vi "Periodic Tasks.vi"(8 "error in":errorcluster) -> ()   [LabVIEW 2018]
doc: "This VI runs in parallel to other tasks. It can contain as many user-defined periodic loops as you need. These can carry out PID or other sorts of timed response."
uses:
  <vilib>/Rock Robotics/WPI/Solenoid/WPI_SolenoidValue.ctl
  <vilib>/Rock Robotics/WPI/ThirdParty/Phoenix-LabVIEW/Motor Controller/Controls/CTRE_Phoenix_MotorControl_ControlMode.ctl
  <vilib>/Rock Robotics/WPI/DriverStation/WPI_DriverStationRobotMode2.ctl
  ca579f97-49ab-43f2-8d57-79325bc44b91.vi
  49744297-d732-4f26-b9df-ea13e04ead65.vi
  0c7d2dc5-c582-4743-8fb3-b9c2bdc871ef.vi
  0ab41fdd-f005-4a41-8abb-d0c1aebc8839.vi
  eb1224c5-d191-4a5a-b208-f0176ff8254b.vi
  4d1e90e2-2e56-4cd0-9c54-8509fccd737b.vi
  fa0b2ed9-014b-4d02-a9e7-965de739ed34.vi
  3bc81077-0bee-49a4-9064-f6dc6ff34700.vi
  c6107473-3bbc-4d68-b130-33bb0f28684e.vi
  bc72f310-a025-467b-8a7d-9af20b832017.vi
  627df16c-e363-45ec-ab0c-cc0e3a3b33f7.vi
  ea05d6e2-4bc2-4863-96e4-0034388c650a.vi
  93672789-ce46-4bc6-a5b5-faff44e817a8.vi
  c8be7294-c6ee-427e-ae78-3199e8744a18.vi
  1c7609ed-6cb5-470b-bbb9-41d14296924d.vi
  50b6936b-a54e-4087-a151-83919d29fb22.vi
  efed0d96-a490-4904-9cbf-ad4873da1ad9.vi
  RobotStates.vi
  Robot Global Data.vi
  <vilib>/Rock Robotics/Network Tables/NT Write Number.vi
  RefNums_DriverStation.vi
  <vilib>/Rock Robotics/WPI/Utilities/WPI_GetSetVariantRefNum.vi
  RefNums_Actuators.vi
  <vilib>/Rock Robotics/WPI/Solenoid/WPI_SolenoidSetEnum.vi
  RefNums_Sensors.vi
  SensorReadings.vi
  Inputs_DriverStation.vi
panel:
  in  "Time in Error Band (ms)":u32=500
  in  "Error Band (in)":dbl=1.0
  in  "Max Down Power":dbl=-0.5 format="%#_13g"
  out "Sensor Loop (ms)":u32
  in  "Enable Plotting":bool
  out "Control Loop Time (ms)":u32
  out "PID Tracking":cluster{"Goal Wheel Position":dbl, dbl}(graph)={"Goal Wheel Position"=0.0, -90.17571233858979}
  out "Contribution Tracking":cluster{dbl, dbl, dbl}(graph)
  in  "N-Int":i32=25
  in  "N-Diff":i32=20
  in  "Kd":dbl=0.01
  in  "Ki":dbl=0.02
  in  "Kp":dbl=0.04
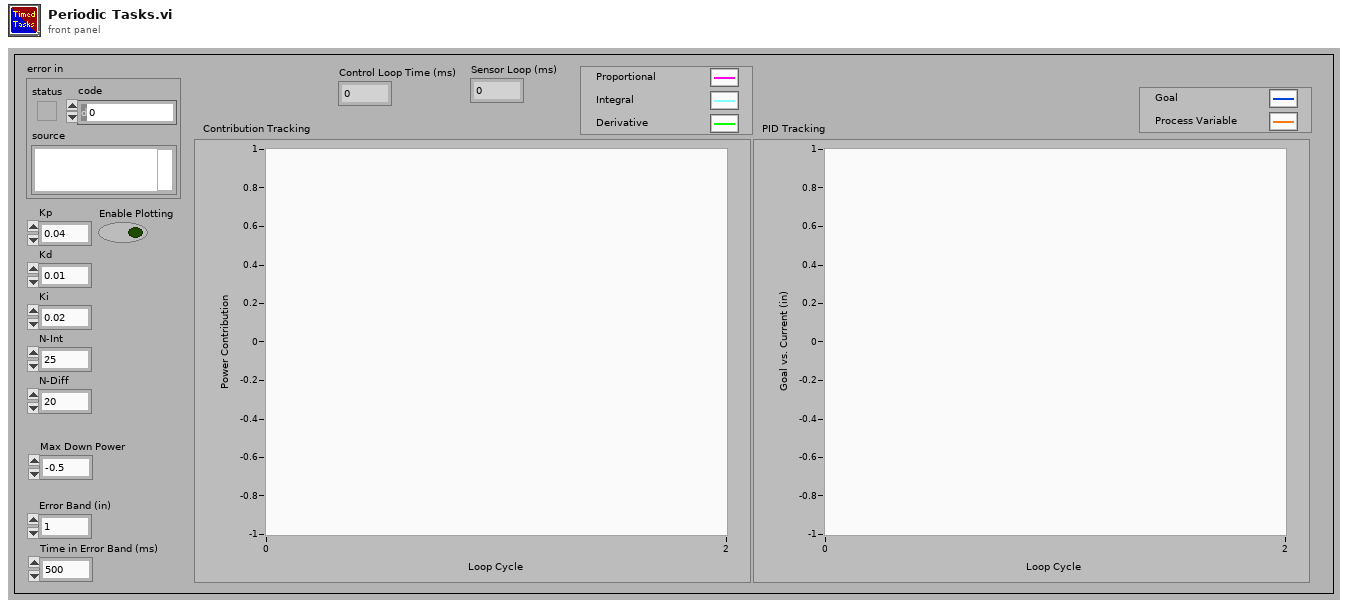
[diagram p1: front panel]
types:
  T1 = typedef "WPI_MotorControlDeviceRef.ctl" = cluster{"DeviceStatus":errorcluster, "Type":T2, "PWM":cluster{"PWM Channel":T3, "DeadBand":T4}, "CAN":cluster{"Device Number":u8, "SetOutput VI Ref":variant, "GetOutput VI Ref":variant, "Enable VI Ref":variant, "Disable VI Ref":variant, "Data":variant}, "Invert":bool, "DIO PWM":cluster{"PWM \"Enable\" Channel":T3, "DIOChannel":T5, "PWM Rate":dbl}}
  T2 = typedef "WPI_MotorControlType.ctl" = enum16{"PWM", "CAN", "DIO PWM"}
  T3 = typedef "FPGA_DIOPWMChannel.ctl" = enum8{"PWM 0", "PWM 1", "PWM 2", "PWM 3", "PWM 4", "PWM 5", "PWM 6", "PWM 7", "PWM 8", "PWM 9", "PWM MXP 0", "PWM MXP 1", "PWM MXP 2", "PWM MXP 3", "PWM MXP 4", "PWM MXP 5", "PWM MXP 6", "PWM MXP 7", "PWM MXP 8", "PWM MXP 9", "Invalid"}
  T4 = typedef "WPI_PWMDeadband.ctl" = cluster{"Name":string, "maxPositivePwm":i32, "minPositivePwm":i32, "centerPwm":i32, "maxNegativePwm":i32, "minNegativePwm":i32, "angularRange":u16}
  T5 = typedef "FPGA_DIOChannel.ctl" = enum8{"DIO 0", "DIO 1", "DIO 2", "DIO 3", "DIO 4", "DIO 5", "DIO 6", "DIO 7", "DIO 8", "DIO 9", "DIO MXP 0", "DIO MXP 1", "DIO MXP 2", "DIO MXP 3", "DIO MXP 4", "DIO MXP 5", "DIO MXP 6", "DIO MXP 7", "DIO MXP 8", "DIO MXP 9", "DIO MXP 10", "DIO MXP 11", "DIO MXP 12", "DIO MXP 13", "DIO MXP 14", "DIO MXP 15", "SPI Port CS1", "SPI Port CS2", "SPI Port CS3", "SPI Port MISO", "SPI Port MOSI", "Invalid"}
  T6 = typedef "WPI_SolenoidDevRef.ctl" = cluster{"DevStatus":errorcluster, "Pneumatics Control Module":u8, "Forward Solenoid Channel":T7, "Reverse Solenoid Channel":T7}
  T7 = typedef "WPI_SolenoidChannel.ctl" = enum8{"Solenoid 0", "Solenoid 1", "Solenoid 2", "Solenoid 3", "Solenoid 4", "Solenoid 5", "Solenoid 6", "Solenoid 7", "Invalid"}
  T8 = typedef "WPI_ServoDeviceRef.ctl" = cluster{"DeviceStatus":errorcluster, "PWM Channel":T3, "DeadBand":T4}
  T9 = typedef "WPI_RobotDriveDevRef.ctl" = cluster{"DevStatus":errorcluster, "Motors[]":T1[], "Square Inputs":bool, "Max Output":dbl}
  T10 = typedef "WPI_JoystickDevRef.ctl" = cluster{"Device":T11}
  T11 = typedef "WPI_JoystickDeviceEnum.ctl" = enum16{"USB 0", "USB 1", "USB 2", "USB 3", "USB 4", "USB 5"}
  T12 = typedef "WPI_CompressorDevRef.ctl" = cluster{"DevStatus":errorcluster, "Pneumatics Control Module":u8}
  T13 = typedef "WPI_AccelerometerDevRef.ctl" = cluster{"DevStatus":errorcluster, "Scaling":T14, "Analog Channels":T15, "I2C Bus":T17, "SPI Bus":T18, "Accel Range":T19, "ADXL Axes":T20, "Handle":i32, "Device Address":u8, "Accel Type":enum16{"Analog", "ADXL345 I2C", "ADXL345 SPI", "Internal", "ADXL362 SPI"}}
  T14 = typedef "WPI_AccelerometerScaling.ctl" = cluster{"Gain (VoltsPerG)":dbl, "Center Voltage":dbl}
  T15 = typedef "WPI_AccelerometerAnalogChannels.ctl" = cluster{"X-Axis":T16, "Y-Axis":T16, "Z-Axis":T16}
  T16 = typedef "FPGA_AIChannel.ctl" = enum8{"AI 0", "AI 1", "AI 2", "AI 3", "AI MXP 0", "AI MXP 1", "AI MXP 2", "AI MXP 3", "Invalid"}
  T17 = typedef "i2c_bus.ctl" = enum16{"I2C On-Board", "I2C MXP", "Invalid"}
  T18 = typedef "spi_bus.ctl" = enum16{"SPI On-Board, CS0", "SPI On-Board, CS1", "SPI On-Board, CS2", "SPI On-Board, CS3", "SPI MXP", "Invalid"}
  T19 = typedef "ADXL345 Range.ctl" = u8
  T20 = typedef "WPI_AccelerometerADXL345 Axes.ctl" = cluster{"X-Axis":bool, "Y-Axis":bool, "Z-Axis":bool}
  T21 = typedef "WPI_AnalogChannelDevRef.ctl" = cluster{"DevStatus":errorcluster, "Analog Channel":T16}
  T22 = typedef "WPI_DriverStationRobotMode2.ctl" = enum16{"Autonomous Disabled", "Autonomous Enabled", "Teleop Disabled", "Teleop Enabled", "Disconnected", "Finish", "Test Disabled", "Test Enabled", "Emergency Stopped"}
  T23 = typedef "CTRE_Phoenix_MotorControl_ControlMode.ctl" = u16
  T24 = typedef "WPI_SolenoidValue.ctl" = enum16{"Off", "On", "Forward", "Reverse"}
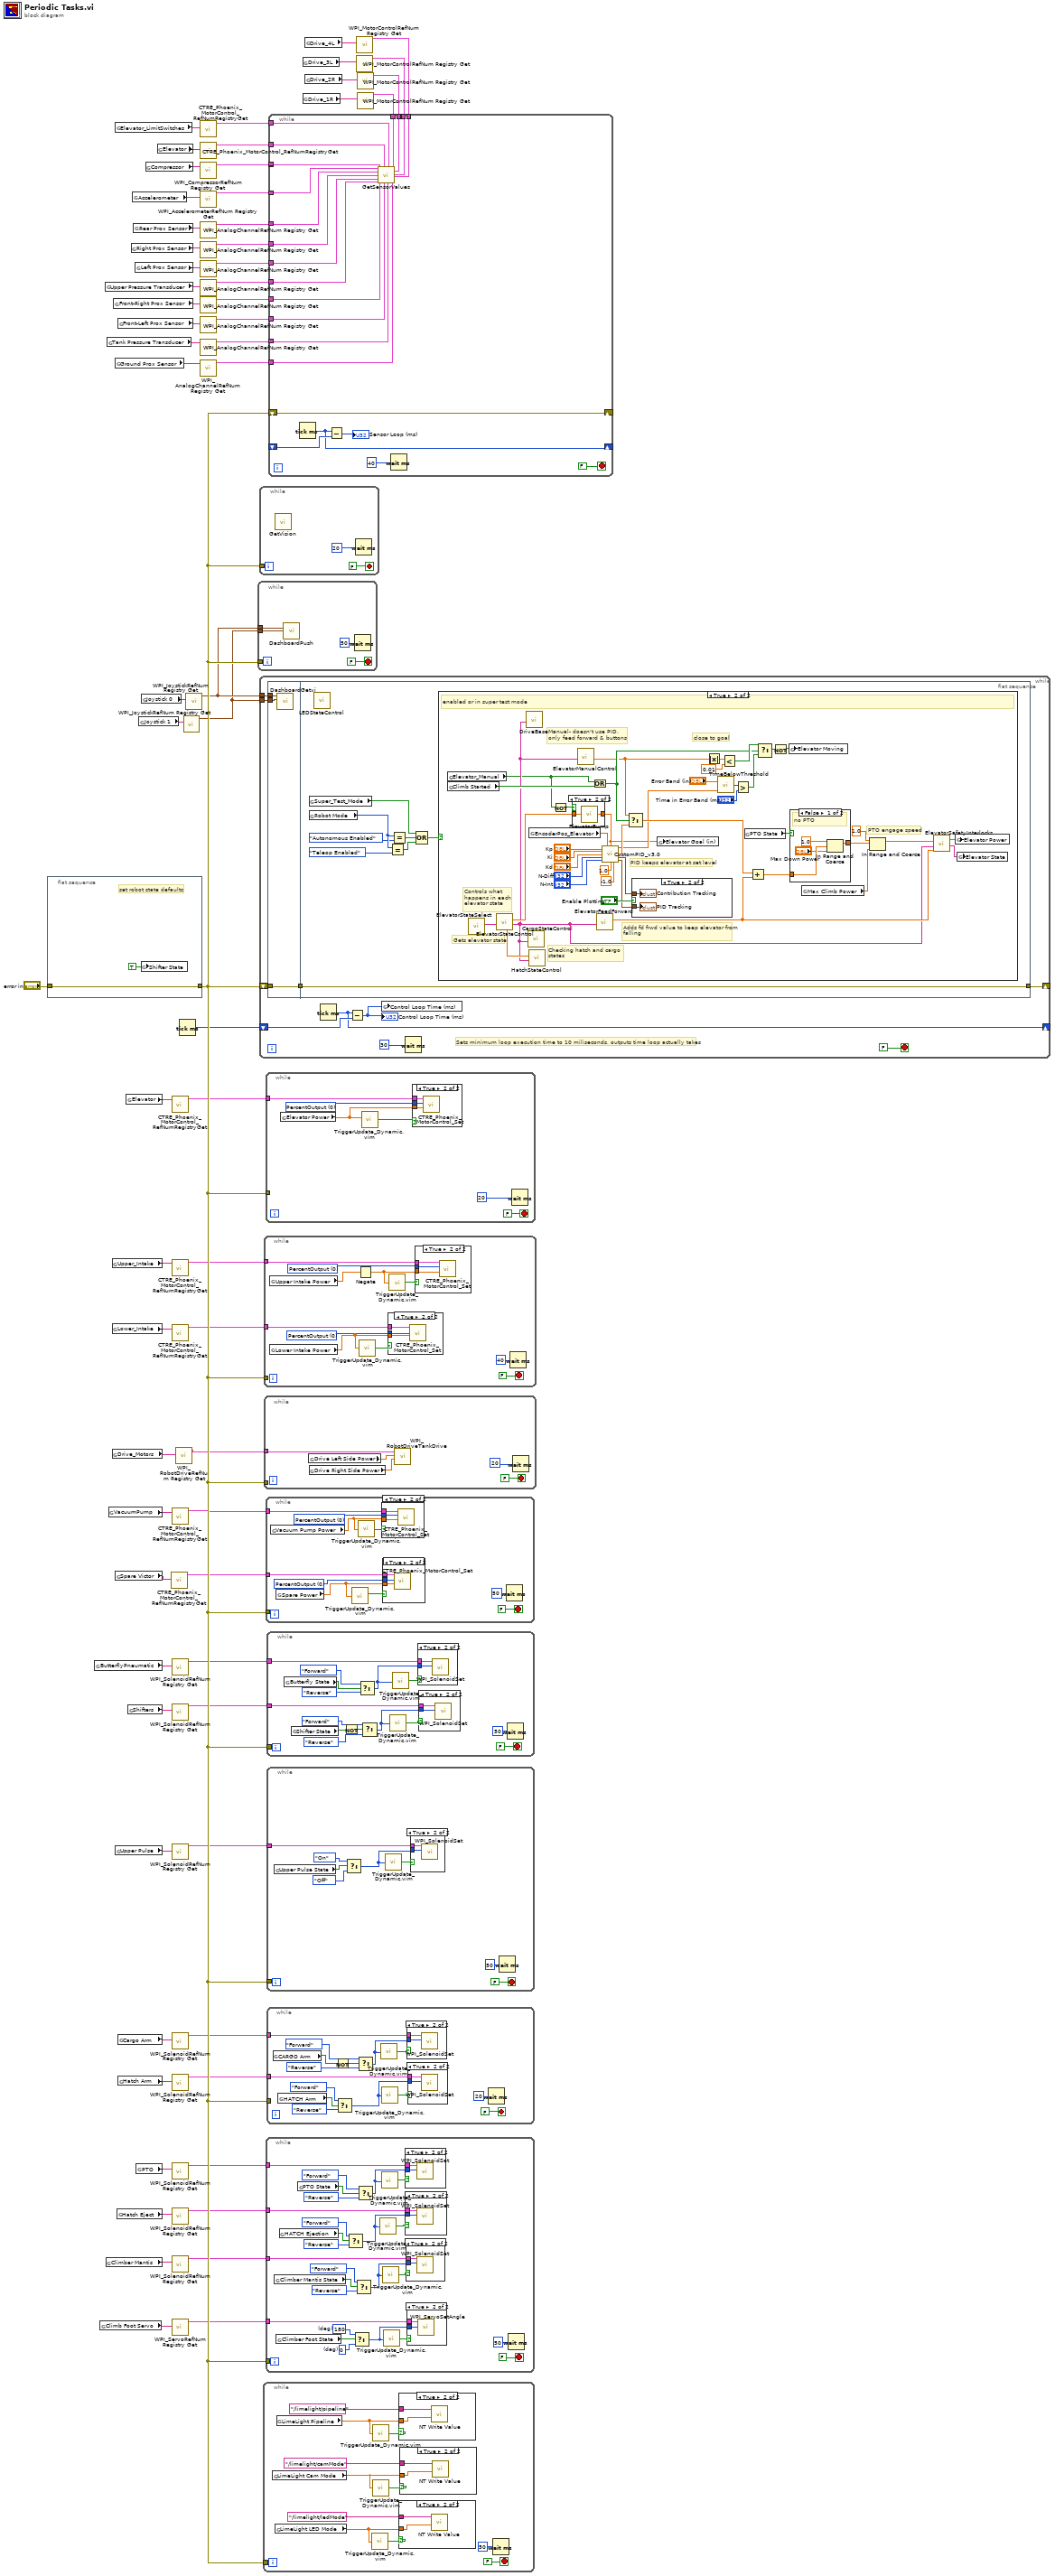
[diagram p0: block diagram]
diagram:
  n1 = flat-sequence {
    tunnel: [w71] -> w69
    tunnel: "error in" -> [w71]
    frame #0 {
      # "set robot state defaults"
      n2 = global write "RobotStates.vi" "Shifter State"(TRUE ("Shifter State")) -> ()
    }
  }
  n3 = global read "RefNums_Actuators.vi" "ButterflyPneumatic"() -> (w66:string)
  n4 = global read "RefNums_Actuators.vi" "Climb Foot Servo"() -> (w1:string)
  n5 = global read "RefNums_Sensors.vi" "Upper Pressure Transducer"() -> (w31:string)
  n6 = global read "RefNums_Actuators.vi" "Climber Mantis"() -> (w46:string)
  n7 = global read "RefNums_Sensors.vi" "Tank Pressure Transducer"() -> (w28:string)
  n8 = global read "RefNums_Actuators.vi" "VacuumPump"() -> (w59:string)
  n9 = global read "RefNums_Actuators.vi" "Upper_Intake"() -> (w56:string)
  n10 = global read "RefNums_Actuators.vi" "Lower_Intake"() -> (w55:string)
  n11 = global read "RefNums_Actuators.vi" "Drive_Motors"() -> (w17:string)
  n12 = global read "RefNums_Sensors.vi" "Front-Right Prox Sensor"() -> (w29:string)
  n13 = global read "RefNums_Actuators.vi" "Elevator_LimitSwitches"() -> (w15:string)
  n14 = global read "RefNums_Sensors.vi" "Ground Prox Sensor"() -> (w4:string)
  n15 = global read "RefNums_Actuators.vi" "Spare Victor"() -> (w52:string)
  n16 = global read "RefNums_Actuators.vi" "Upper Pulse"() -> (w62:string)
  n17 = global read "RefNums_Actuators.vi" "Hatch Eject"() -> (w47:string)
  n18 = global read "RefNums_Sensors.vi" "Front-Left Prox Sensor"() -> (w30:string)
  n19 = global read "RefNums_Actuators.vi" "Cargo Arm"() -> (w58:string)
  n20 = global read "RefNums_Actuators.vi" "Hatch Arm"() -> (w48:string)
  n21 = global read "RefNums_Actuators.vi" "Elevator"() -> (w22:string)
  n22 = global read "RefNums_Actuators.vi" "Shifters"() -> (w64:string)
  n23 = global read "RefNums_Sensors.vi" "Right Prox Sensor"() -> (w35:string)
  n24 = global read "RefNums_Sensors.vi" "Accelerometer"() -> (w7:string)
  n25 = global read "RefNums_Sensors.vi" "Rear Prox Sensor"() -> (w37:string)
  n26 = global read "RefNums_Sensors.vi" "Left Prox Sensor"() -> (w36:string)
  n27 = global read "RefNums_Actuators.vi" "PTO"() -> (w50:string)
  n28 = global read "RefNums_DriverStation.vi" "Joystick 1"() -> (w21:string)
  n29 = global read "RefNums_DriverStation.vi" "Joystick 0"() -> (w67:string)
  n30 = global read "RefNums_Actuators.vi" "Compressor"() -> (w41:string)
  n31 = global read "RefNums_Actuators.vi" "Elevator"() -> (w40:string)
  n32 = call <vilib>:"CTRE_Phoenix_MotorControl_RefNumRegistryGet.vi"("refnum name"=w52) -> ("PhoenixMotorControlDevRef"=w51:T1)  [unwired: 9 in, 1 out]
  n33 = call <vilib>:"CTRE_Phoenix_MotorControl_RefNumRegistryGet.vi"("refnum name"=w22) -> ("PhoenixMotorControlDevRef"=w68:T1)  [unwired: 9 in, 1 out]
  n34 = call <vilib>:"CTRE_Phoenix_MotorControl_RefNumRegistryGet.vi"("refnum name"=w56) -> ("PhoenixMotorControlDevRef"=w54:T1)  [unwired: 9 in, 1 out]
  n35 = call <vilib>:"CTRE_Phoenix_MotorControl_RefNumRegistryGet.vi"("refnum name"=w55) -> ("PhoenixMotorControlDevRef"=w53:T1)  [unwired: 9 in, 1 out]
  n36 = call <vilib>:"CTRE_Phoenix_MotorControl_RefNumRegistryGet.vi"("refnum name"=w59) -> ("PhoenixMotorControlDevRef"=w60:T1)  [unwired: 9 in, 1 out]
  n37 = call <vilib>:"WPI_SolenoidRefNum Registry Get.vi"("refnum name"=w66) -> ("SolenoidDevRef"=w65:T6)  [unwired: 9 in, 1 out]
  n38 = call <vilib>:"WPI_SolenoidRefNum Registry Get.vi"("refnum name"=w64) -> ("SolenoidDevRef"=w63:T6)  [unwired: 9 in, 1 out]
  n39 = call <vilib>:"WPI_SolenoidRefNum Registry Get.vi"("refnum name"=w62) -> ("SolenoidDevRef"=w61:T6)  [unwired: 9 in, 1 out]
  n40 = call <vilib>:"WPI_SolenoidRefNum Registry Get.vi"("refnum name"=w58) -> ("SolenoidDevRef"=w57:T6)  [unwired: 9 in, 1 out]
  n41 = call <vilib>:"WPI_SolenoidRefNum Registry Get.vi"("refnum name"=w48) -> ("SolenoidDevRef"=w45:T6)  [unwired: 9 in, 1 out]
  n42 = call <vilib>:"WPI_SolenoidRefNum Registry Get.vi"("refnum name"=w50) -> ("SolenoidDevRef"=w49:T6)  [unwired: 9 in, 1 out]
  n43 = call <vilib>:"WPI_SolenoidRefNum Registry Get.vi"("refnum name"=w47) -> ("SolenoidDevRef"=w44:T6)  [unwired: 9 in, 1 out]
  n44 = call <vilib>:"WPI_SolenoidRefNum Registry Get.vi"("refnum name"=w46) -> ("SolenoidDevRef"=w43:T6)  [unwired: 9 in, 1 out]
  n45 = call <vilib>:"WPI_ServoRefNum Registry Get.vi"("refnum name"=w1) -> ("ServoDeviceRef"=w2:T8)  [unwired: 9 in, 1 out]
  n46 = call <vilib>:"WPI_RobotDriveRefNum Registry Get.vi"("refnum name"=w17) -> ("RobotDriveDevRef"=w16:T9)  [unwired: 9 in, 1 out]
  n47 = Tick Count (ms)() -> (millisecond timer value=w42:u32)
  n48 = call <vilib>:"WPI_JoystickRefNum Registry Get.vi"("refnum name"=w21) -> ("JoystickDevRef"=w5:T10)  [unwired: 9 in, 1 out]
  n49 = call <vilib>:"WPI_JoystickRefNum Registry Get.vi"("refnum name"=w67) -> ("JoystickDevRef"=w23:T10)  [unwired: 9 in, 1 out]
  n50 = call <vilib>:"CTRE_Phoenix_MotorControl_RefNumRegistryGet.vi"("refnum name"=w15) -> ("PhoenixMotorControlDevRef"=w14:T1)  [unwired: 9 in, 1 out]
  n51 = call <vilib>:"CTRE_Phoenix_MotorControl_RefNumRegistryGet.vi"("refnum name"=w40) -> ("PhoenixMotorControlDevRef"=w39:T1)  [unwired: 9 in, 1 out]
  n52 = call <vilib>:"WPI_CompressorRefNum Registry Get.vi"("refnum name"=w41) -> ("CompressorDevRef"=w38:T12)  [unwired: 9 in, 1 out]
  n53 = call <vilib>:"WPI_AccelerometerRefNum Registry Get.vi"("refnum name"=w7) -> ("AccelerometerDevRef"=w6:T13)  [unwired: 9 in, 1 out]
  n54 = call <vilib>:"WPI_AnalogChannelRefNum Registry Get.vi"("refnum name"=w37) -> ("AIDeviceRef"=w34:T21)  [unwired: 9 in, 1 out]
  n55 = call <vilib>:"WPI_AnalogChannelRefNum Registry Get.vi"("refnum name"=w35) -> ("AIDeviceRef"=w33:T21)  [unwired: 9 in, 1 out]
  n56 = call <vilib>:"WPI_AnalogChannelRefNum Registry Get.vi"("refnum name"=w36) -> ("AIDeviceRef"=w32:T21)  [unwired: 9 in, 1 out]
  n57 = call <vilib>:"WPI_AnalogChannelRefNum Registry Get.vi"("refnum name"=w31) -> ("AIDeviceRef"=w27:T21)  [unwired: 9 in, 1 out]
  n58 = call <vilib>:"WPI_AnalogChannelRefNum Registry Get.vi"("refnum name"=w29) -> ("AIDeviceRef"=w26:T21)  [unwired: 9 in, 1 out]
  n59 = call <vilib>:"WPI_AnalogChannelRefNum Registry Get.vi"("refnum name"=w30) -> ("AIDeviceRef"=w25:T21)  [unwired: 9 in, 1 out]
  n60 = call <vilib>:"WPI_AnalogChannelRefNum Registry Get.vi"("refnum name"=w28) -> ("AIDeviceRef"=w24:T21)  [unwired: 9 in, 1 out]
  n61 = call <vilib>:"WPI_AnalogChannelRefNum Registry Get.vi"("refnum name"=w4) -> ("AIDeviceRef"=w3:T21)  [unwired: 9 in, 1 out]
  n62 = while {
    tunnel: w23 -> [w74]
    tunnel: w69 -> [_]
    tunnel: w5 -> [w72]
    stop <- FALSE stop-if-true
    n63 = call "DashboardPush.vi"("Joystick 0 Ref"=w74, "Joystick 1 Ref"=w72) -> ()  [unwired: 14 in]
    n64 = Wait (ms)(milliseconds to wait=u32 50) -> ()  [unwired: 1 out]
  }
  n65 = while {
    tunnel: w69 -> [_]
    stop <- FALSE stop-if-true
    n66 = call "GetVision.vi"() -> ()  [unwired: 12 in]
    n67 = Wait (ms)(milliseconds to wait=u32 20) -> ()  [unwired: 1 out]
  }
  n68 = while {
    shift-right: [w84] -> _
    shift-left: w69 -> [w86]
    tunnel: w23 -> [w83]
    shift-right: [w81] -> _
    shift-left: w42 -> [w82]
    tunnel: w5 -> [w79]
    stop <- FALSE stop-if-true
    # "Sets minimum loop execution time to 10 miliseconds, outputs time loop actually takes"
    n69 = flat-sequence {
      tunnel: w83 -> [w90]
      tunnel: w86 -> [w89]
      tunnel: [w89] -> w85
      tunnel: w79 -> [w88]
      tunnel: w85 -> [w98]
      tunnel: [w98] -> w84
      frame #0 {
        n70 = call "DashboardGetvi.vi"("Joystick 2"=w88, "Joystick 1"=w90) -> ()  [unwired: 8 in]
      }
      frame #1 {
        n71 = global read "Inputs_DriverStation.vi" "Super_Test_Mode"() -> (w91:bool)
        n72 = global read "Robot Global Data.vi" "Robot Mode"() -> (w95:T22)
        n73 = call "LEDStateControl.vi"() -> ()  [unwired: 12 in]
        n74 = Equal?(x=w95, y=WPI_DriverStationRobotMode2."Teleop Enabled") -> (x = y?=w96:bool)
        n75 = Equal?(x=w95, y=WPI_DriverStationRobotMode2."Autonomous Enabled") -> (x = y?=w97:bool)
        n76 = Compound Arithmetic op=OR(w91, w97, w96) -> (w92:bool)
        n77 = case shown="True" w92 {
          frame False {
            # "disabled and not in super test mode"
          }
          frame True {
            # "PTO engage speed"
            # "close to goal"
            # "PID keeps elevator at set level"
            # "Manual- doesn't use PID,\nonly feed forward & buttons"
            # "Adds fd frwd value to keep elevator from falling"
            # "Checking hatch and cargo \nstates"
            # "Controls what\nhappens in each \nelevator state"
            # "Gets elevator state"
            # "enabled or in super test mode"
            n78 = global read "Inputs_DriverStation.vi" "Elevator_Manual"() -> (w99:bool)
            n79 = global read "RobotStates.vi" "Climb Started"() -> (w124:bool)
            n80 = call "ElevatorStateSelect.vi"() -> ("Elevator State"=w137:string)  [unwired: 11 in]
            n81 = call "ElevatorStateControl.vi"("Elevator State"=w137) -> ("Elevator State Out"=w107:string, "Target Elevator Position"=w140:dbl, "Target Vacuum Pump Power"=w125:dbl)  [unwired: 8 in]
            n82 = call "DriveBase.vi"("Elevator State"=w107) -> ()  [unwired: 11 in]
            n83 = call "CargoStateControl.vi"("Elevator State"=w107) -> ()  [unwired: 11 in]
            n84 = call "HatchStateControl.vi"("Elevator State"=w107, "Vacuum Pump Power"=w125) -> ()  [unwired: 10 in]
            n85 = global read "SensorReadings.vi" "EncoderPos_Elevator"() -> (w135:dbl)
            n86 = Not(x=w99) -> (.not. x?=w100:bool)
            n87 = case shown="True" w100 {
              tunnel: w140 -> [w141 w143]
              tunnel: [w141 w142] -> w101
              frame False {
              }
              frame True {
                n88 = call "ElevatorBump.vi"("Elevator Goal In (in)"=w143) -> ("Elevator Goal Out (in)"=w142:dbl)
              }
            }
            n89 = call "ElevatorManualControl.vi"("Elevator State"=w107) -> ("Manual Contribution"=w108:dbl)  [unwired: 10 in]
            n90 = Or(x=w99, y=w124) -> (x .or. y?=w110:bool)
            n91 = call "ElevatorFeedForward.vi"("Elevator State"=w107) -> ("Feed Forward Contribution"=w121:dbl)  [unwired: 10 in]
            n92 = call "CustomPID_v3.0.vi"("Kp"="Kp", "Process Variable"=w135, "Goal"=w101, "Ki"="Ki", "Kd"="Kd", "N-Diff"="N-Diff", "N-Int"="N-Int", "Max Ouput"=1.0, "Min Output"=-1.0) -> ("Current Error"=w116:dbl, "Command"=w136:dbl, "Contribution Tracking"=w127:cluster{dbl, dbl, dbl}, "PID Tracking"=w126:cluster{"Goal Wheel Position":dbl, dbl})  [unwired: 3 in]
            n93 = Select(t=w108, s=w110, f=w136) -> (s? t:f=w138:dbl)
            n94 = case shown="True" "Enable Plotting" {
              tunnel: w127 -> [_ w153]
              tunnel: w126 -> [_ w152]
              frame False {
              }
              frame True {
                "Contribution Tracking" <- w153
                "PID Tracking" <- w152
              }
            }
            n95 = global write "RobotStates.vi" "Elevator Goal (in)"(w101) -> ()
            n96 = Absolute Value(x=w108) -> (abs(x)=w115:dbl)
            n97 = call "TimeBelowThreshold.vi"("Current Value"=w116, "Threshold"="Error Band (in)") -> ("Time Below"=w118:u32)  [unwired: 3 in]
            n98 = Less?(x=w115, y=0.01) -> (x < y?=w114:bool)
            n99 = Greater?(x=w118, y="Time in Error Band (ms)") -> (0:w109:bool)
            n100 = global read "RobotStates.vi" "PTO State"() -> (w106:bool)
            n101 = Add(x=w138, y=w121) -> (x+y=w120:dbl)
            n102 = Select(t=w114, s=w110, f=w109) -> (s? t:f=w113:bool)
            n103 = Not(x=w113) -> (.not. x?=w112:bool)
            n104 = global write "RobotStates.vi" "Elevator Moving"(w112) -> ()
            n105 = case shown="False" w106 {
              tunnel: w120 -> [w147 w150]
              tunnel: [w144 w151] -> w104
              frame False {
                # "no PTO"
                n106 = In Range and Coerce(upper limit=1.0, x=w147, lower limit="Max Down Power") -> (coerced(x)=w144:dbl)  [unwired: 1 out]
              }
              frame True {
                # "PTO"
                n107 = In Range and Coerce(upper limit=1.0, x=w150, lower limit=-1.0) -> (coerced(x)=w151:dbl)  [unwired: 1 out]
              }
            }
            n108 = global read "RobotStates.vi" "Max Climb Power"() -> (w102:dbl)
            n109 = In Range and Coerce(upper limit=1.0, x=w104, lower limit=w102) -> (coerced(x)=w105:dbl)  [unwired: 1 out]
            n110 = call "ElevatorSafetyInterlocks.vi"("Feed Forward Contribution"=w121, "Elevator State In"=w107, "Elevator Power In"=w105) -> ("Elevator State Out"=w122:string, "Elevator Power Out"=w123:dbl)  [unwired: 7 in]
            n111 = global write "RobotStates.vi" "Elevator Power"(w123) -> ()
            n112 = global write "RobotStates.vi" "Elevator State"(w122) -> ()
          }
        }
      }
    }
    n113 = Tick Count (ms)() -> (millisecond timer value=w81:u32)
    n114 = Subtract(x=w81, y=w82) -> (x-y=w80:u32)
    "Control Loop Time (ms)" <- w80
    n115 = global write "SensorReadings.vi" "Control Loop Time (ms)"(w80) -> ()
    n116 = Wait (ms)(milliseconds to wait=u32 30) -> ()  [unwired: 1 out]
  }
  n117 = while {
    tunnel: w69 -> [_]
    stop <- FALSE stop-if-true
    n118 = global read "RobotStates.vi" "LimeLight Cam Mode"() -> (w157:dbl)
    n119 = global read "RobotStates.vi" "LimeLight LED Mode"() -> (w160:dbl)
    n120 = global read "RobotStates.vi" "LimeLight Pipeline"() -> (w154:dbl)
    n121 = call "TriggerUpdate_Dynamic.vim"("Trigger"=w160) -> ("Update"=w162:bool)
    n122 = call "TriggerUpdate_Dynamic.vim"("Trigger"=w154) -> ("Update"=w156:bool)
    n123 = call "TriggerUpdate_Dynamic.vim"("Trigger"=w157) -> ("Update"=w159:bool)
    n124 = case shown="True" w162 {
      tunnel: "/limelight/ledMode" ("Name") -> [_ w170]
      tunnel: w160 -> [_ w169]
      frame False {
      }
      frame True {
        n125 = call-poly <vilib>:"NT Write Value.vi"("Numeric"=w169, "Name"=w170) -> ()  [unwired: 9 in, 1 out]
      }
    }
    n126 = case shown="True" w156 {
      tunnel: "/limelight/pipeline" ("Name") -> [_ w166]
      tunnel: w154 -> [_ w165]
      frame False {
      }
      frame True {
        n127 = call-poly <vilib>:"NT Write Value.vi"("Numeric"=w165, "Name"=w166) -> ()  [unwired: 9 in, 1 out]
      }
    }
    n128 = case shown="True" w159 {
      tunnel: "/limelight/camMode" ("Name") -> [_ w168]
      tunnel: w157 -> [_ w167]
      frame False {
      }
      frame True {
        n129 = call-poly <vilib>:"NT Write Value.vi"("Numeric"=w167, "Name"=w168) -> ()  [unwired: 9 in, 1 out]
      }
    }
    n130 = Wait (ms)(milliseconds to wait=u32 50) -> ()  [unwired: 1 out]
  }
  n131 = while {
    tunnel: w54 -> [w181]
    tunnel: w53 -> [w180]
    tunnel: w69 -> [_]
    stop <- FALSE stop-if-true
    w178 = T23 0 items=["PercentOutput"=0, "Position"=1, "Velocity"=2, "Current"=3, "Follower"=5, "MotionProfile"=6, "MotionMagic"=7, "MotionProfileArc"=10, "Disabled"=15] ("Control Mode")
    w179 = T23 0 items=["PercentOutput"=0, "Position"=1, "Velocity"=2, "Current"=3, "Follower"=5, "MotionProfile"=6, "MotionMagic"=7, "MotionProfileArc"=10, "Disabled"=15] ("Control Mode")
    n132 = global read "RobotStates.vi" "Upper Intake Power"() -> (w175:dbl)
    n133 = global read "RobotStates.vi" "Lower Intake Power"() -> (w173:dbl)
    n134 = Negate(x=w175) -> (-x=w171:dbl)
    n135 = call "TriggerUpdate_Dynamic.vim"("Trigger"=w173) -> ("Update"=w172:bool)
    n136 = case shown="True" w172 {
      tunnel: w180 -> [_ w184]
      tunnel: w178 -> [_ w183]
      tunnel: w173 -> [_ w182]
      frame False {
      }
      frame True {
        n137 = call <vilib>:"CTRE_Phoenix_MotorControl_Set.vi"("Output"=w182, "Control Mode"=w183, "PhoenixMotorControlDevRef"=w184) -> ()  [unwired: 7 in, 2 out]
      }
    }
    n138 = call "TriggerUpdate_Dynamic.vim"("Trigger"=w171) -> ("Update"=w174:bool)
    n139 = case shown="True" w174 {
      tunnel: w181 -> [_ w187]
      tunnel: w179 -> [_ w186]
      tunnel: w171 -> [_ w185]
      frame False {
      }
      frame True {
        n140 = call <vilib>:"CTRE_Phoenix_MotorControl_Set.vi"("Output"=w185, "Control Mode"=w186, "PhoenixMotorControlDevRef"=w187) -> ()  [unwired: 7 in, 2 out]
      }
    }
    n141 = Wait (ms)(milliseconds to wait=u32 40) -> ()  [unwired: 1 out]
  }
  n142 = while {
    tunnel: w16 -> [w192]
    tunnel: w69 -> [_]
    stop <- FALSE stop-if-true
    n143 = global read "RobotStates.vi" "Drive Left Side Power"() -> (w190:dbl)
    n144 = global read "RobotStates.vi" "Drive Right Side Power"() -> (w189:dbl)
    n145 = call <vilib>:"WPI_RobotDriveTankDrive.vi"("Right axis value"=w189, "Left axis value"=w190, "RobotDriveDevRef"=w192) -> ()  [unwired: 6 in, 3 out]
    n146 = Wait (ms)(milliseconds to wait=u32 20) -> ()  [unwired: 1 out]
  }
  n147 = while {
    tunnel: w69 -> [_]
    tunnel: w68 -> [w197]
    stop <- FALSE stop-if-true
    w196 = T23 0 items=["PercentOutput"=0, "Position"=1, "Velocity"=2, "Current"=3, "Follower"=5, "MotionProfile"=6, "MotionMagic"=7, "MotionProfileArc"=10, "Disabled"=15] ("Control Mode")
    n148 = global read "RobotStates.vi" "Elevator Power"() -> (w195:dbl)
    n149 = call "TriggerUpdate_Dynamic.vim"("Trigger"=w195) -> ("Update"=w194:bool)
    n150 = case shown="True" w194 {
      tunnel: w197 -> [_ w201]
      tunnel: w196 -> [_ w200]
      tunnel: w195 -> [_ w199]
      frame False {
      }
      frame True {
        n151 = call <vilib>:"CTRE_Phoenix_MotorControl_Set.vi"("Output"=w199, "Control Mode"=w200, "PhoenixMotorControlDevRef"=w201) -> ()  [unwired: 7 in, 2 out]
      }
    }
    n152 = Wait (ms)(milliseconds to wait=u32 20) -> ()  [unwired: 1 out]
  }
  n153 = while {
    tunnel: w60 -> [w211]
    tunnel: w51 -> [w210]
    tunnel: w69 -> [_]
    stop <- FALSE stop-if-true
    w202 = T23 0 items=["PercentOutput"=0, "Position"=1, "Velocity"=2, "Current"=3, "Follower"=5, "MotionProfile"=6, "MotionMagic"=7, "MotionProfileArc"=10, "Disabled"=15] ("Control Mode")
    w209 = T23 0 items=["PercentOutput"=0, "Position"=1, "Velocity"=2, "Current"=3, "Follower"=5, "MotionProfile"=6, "MotionMagic"=7, "MotionProfileArc"=10, "Disabled"=15] ("Control Mode")
    n154 = global read "RobotStates.vi" "Vacuum Pump Power"() -> (w206:dbl)
    n155 = global read "RobotStates.vi" "Spare Power"() -> (w204:dbl)
    n156 = call "TriggerUpdate_Dynamic.vim"("Trigger"=w204) -> ("Update"=w203:bool)
    n157 = call "TriggerUpdate_Dynamic.vim"("Trigger"=w206) -> ("Update"=w205:bool)
    n158 = case shown="True" w205 {
      tunnel: w211 -> [_ w217]
      tunnel: w209 -> [_ w216]
      tunnel: w206 -> [_ w215]
      frame False {
      }
      frame True {
        n159 = call <vilib>:"CTRE_Phoenix_MotorControl_Set.vi"("Output"=w215, "Control Mode"=w216, "PhoenixMotorControlDevRef"=w217) -> ()  [unwired: 7 in, 2 out]
      }
    }
    n160 = case shown="True" w203 {
      tunnel: w210 -> [_ w214]
      tunnel: w202 -> [_ w213]
      tunnel: w204 -> [_ w212]
      frame False {
      }
      frame True {
        n161 = call <vilib>:"CTRE_Phoenix_MotorControl_Set.vi"("Output"=w212, "Control Mode"=w213, "PhoenixMotorControlDevRef"=w214) -> ()  [unwired: 7 in, 2 out]
      }
    }
    n162 = Wait (ms)(milliseconds to wait=u32 50) -> ()  [unwired: 1 out]
  }
  n163 = while {
    tunnel: w49 -> [w243]
    tunnel: w44 -> [w242]
    tunnel: w43 -> [w241]
    tunnel: w69 -> [_]
    tunnel: w2 -> [w222]
    stop <- FALSE stop-if-true
    w219 = 180  # (deg)
    w221 = 0  # (deg)
    n164 = global read "RobotStates.vi" "Climber Mantis State"() -> (w236:bool)
    n165 = global read "RobotStates.vi" "Climber Foot State"() -> (w218:bool)
    n166 = global read "RobotStates.vi" "HATCH Ejection"() -> (w238:bool)
    n167 = global read "RobotStates.vi" "PTO State"() -> (w224:bool)
    n168 = Select(t=WPI_SolenoidValue."Forward" ("Value"), s=w238, f=WPI_SolenoidValue."Reverse") -> (s? t:f=w228:T24)
    n169 = Select(t=w219, s=w218, f=w221) -> (s? t:f=w220:i32)
    n170 = Select(t=WPI_SolenoidValue."Forward" ("Value"), s=w236, f=WPI_SolenoidValue."Reverse") -> (s? t:f=w226:T24)
    n171 = Select(t=WPI_SolenoidValue."Forward" ("Value"), s=w224, f=WPI_SolenoidValue."Reverse") -> (s? t:f=w230:T24)
    n172 = call "TriggerUpdate_Dynamic.vim"("Trigger"=w228) -> ("Update"=w227:bool)
    n173 = call "TriggerUpdate_Dynamic.vim"("Trigger"=w230) -> ("Update"=w229:bool)
    n174 = call "TriggerUpdate_Dynamic.vim"("Trigger"=w226) -> ("Update"=w225:bool)
    n175 = call "TriggerUpdate_Dynamic.vim"("Trigger"=w220) -> ("Update"=w223:bool)
    n176 = case shown="True" w229 {
      tunnel: w243 -> [_ w251]
      tunnel: w230 -> [_ w250]
      frame False {
      }
      frame True {
        n177 = call-poly <vilib>:"WPI_SolenoidSet.vi"("Value"=w250, "SolenoidDevRef"=w251) -> ()  [unwired: 8 in, 2 out]
      }
    }
    n178 = case shown="True" w227 {
      tunnel: w242 -> [_ w249]
      tunnel: w228 -> [_ w248]
      frame False {
      }
      frame True {
        n179 = call-poly <vilib>:"WPI_SolenoidSet.vi"("Value"=w248, "SolenoidDevRef"=w249) -> ()  [unwired: 8 in, 2 out]
      }
    }
    n180 = case shown="True" w225 {
      tunnel: w241 -> [_ w247]
      tunnel: w226 -> [_ w246]
      frame False {
      }
      frame True {
        n181 = call-poly <vilib>:"WPI_SolenoidSet.vi"("Value"=w246, "SolenoidDevRef"=w247) -> ()  [unwired: 8 in, 2 out]
      }
    }
    n182 = case shown="True" w223 {
      tunnel: w220 -> [_ w244]
      tunnel: w222 -> [_ w245]
      frame False {
      }
      frame True {
        n183 = call <vilib>:"WPI_ServoSetAngle.vi"("Angle"=w244, "ServoDeviceRef"=w245) -> ()  [unwired: 8 in, 2 out]
      }
    }
    n184 = Wait (ms)(milliseconds to wait=u32 50) -> ()  [unwired: 1 out]
  }
  n185 = while {
    tunnel: w57 -> [w266]
    tunnel: w45 -> [w265]
    tunnel: w69 -> [_]
    stop <- FALSE stop-if-true
    n186 = global read "RobotStates.vi" "CARGO Arm"() -> (w264:bool)
    n187 = global read "RobotStates.vi" "HATCH Arm"() -> (w261:bool)
    n188 = Not(x=w264) -> (.not. x?=w252:bool)
    n189 = Select(t=WPI_SolenoidValue."Forward" ("Value"), s=w261, f=WPI_SolenoidValue."Reverse") -> (s? t:f=w254:T24)
    n190 = Select(t=WPI_SolenoidValue."Forward" ("Value"), s=w252, f=WPI_SolenoidValue."Reverse") -> (s? t:f=w256:T24)
    n191 = call "TriggerUpdate_Dynamic.vim"("Trigger"=w256) -> ("Update"=w255:bool)
    n192 = call "TriggerUpdate_Dynamic.vim"("Trigger"=w254) -> ("Update"=w253:bool)
    n193 = case shown="True" w255 {
      tunnel: w266 -> [_ w270]
      tunnel: w256 -> [_ w269]
      frame False {
      }
      frame True {
        n194 = call-poly <vilib>:"WPI_SolenoidSet.vi"("Value"=w269, "SolenoidDevRef"=w270) -> ()  [unwired: 8 in, 2 out]
      }
    }
    n195 = case shown="True" w253 {
      tunnel: w265 -> [_ w268]
      tunnel: w254 -> [_ w267]
      frame False {
      }
      frame True {
        n196 = call-poly <vilib>:"WPI_SolenoidSet.vi"("Value"=w267, "SolenoidDevRef"=w268) -> ()  [unwired: 8 in, 2 out]
      }
    }
    n197 = Wait (ms)(milliseconds to wait=u32 20) -> ()  [unwired: 1 out]
  }
  n198 = while {
    tunnel: w65 -> [w285]
    tunnel: w63 -> [w284]
    tunnel: w69 -> [_]
    stop <- FALSE stop-if-true
    n199 = global read "RobotStates.vi" "Butterfly State"() -> (w281:bool)
    n200 = global read "RobotStates.vi" "Shifter State"() -> (w280:bool)
    n201 = Not(x=w280) -> (.not. x?=w271:bool)
    n202 = Select(t=WPI_SolenoidValue."Forward" ("Value"), s=w281, f=WPI_SolenoidValue."Reverse") -> (s? t:f=w275:T24)
    n203 = Select(t=WPI_SolenoidValue."Forward" ("Value"), s=w271, f=WPI_SolenoidValue."Reverse") -> (s? t:f=w273:T24)
    n204 = call "TriggerUpdate_Dynamic.vim"("Trigger"=w273) -> ("Update"=w272:bool)
    n205 = call "TriggerUpdate_Dynamic.vim"("Trigger"=w275) -> ("Update"=w274:bool)
    n206 = case shown="True" w274 {
      tunnel: w285 -> [_ w289]
      tunnel: w275 -> [_ w288]
      frame False {
      }
      frame True {
        n207 = call-poly <vilib>:"WPI_SolenoidSet.vi"("Value"=w288, "SolenoidDevRef"=w289) -> ()  [unwired: 8 in, 2 out]
      }
    }
    n208 = case shown="True" w272 {
      tunnel: w284 -> [_ w287]
      tunnel: w273 -> [_ w286]
      frame False {
      }
      frame True {
        n209 = call-poly <vilib>:"WPI_SolenoidSet.vi"("Value"=w286, "SolenoidDevRef"=w287) -> ()  [unwired: 8 in, 2 out]
      }
    }
    n210 = Wait (ms)(milliseconds to wait=u32 50) -> ()  [unwired: 1 out]
  }
  n211 = while {
    tunnel: w61 -> [w297]
    tunnel: w69 -> [_]
    stop <- FALSE stop-if-true
    n212 = global read "RobotStates.vi" "Upper Pulse State"() -> (w296:bool)
    n213 = Select(t=WPI_SolenoidValue."On" ("Value"), s=w296, f=WPI_SolenoidValue."Off") -> (s? t:f=w291:T24)
    n214 = call "TriggerUpdate_Dynamic.vim"("Trigger"=w291) -> ("Update"=w290:bool)
    n215 = case shown="True" w290 {
      tunnel: w297 -> [_ w299]
      tunnel: w291 -> [_ w298]
      frame False {
      }
      frame True {
        n216 = call-poly <vilib>:"WPI_SolenoidSet.vi"("Value"=w298, "SolenoidDevRef"=w299) -> ()  [unwired: 8 in, 2 out]
      }
    }
    n217 = Wait (ms)(milliseconds to wait=u32 50) -> ()  [unwired: 1 out]
  }
  n218 = global read "RefNums_Actuators.vi" "Drive_3L"() -> (w18:string)
  n219 = global read "RefNums_Actuators.vi" "Drive_1R"() -> (w12:string)
  n220 = global read "RefNums_Actuators.vi" "Drive_4L"() -> (w19:string)
  n221 = global read "RefNums_Actuators.vi" "Drive_2R"() -> (w13:string)
  n222 = call <vilib>:"WPI_MotorControlRefNum Registry Get.vi"("refnum name"=w19) -> ("MotorControlDevRef"=w8:T1)  [unwired: 9 in, 1 out]
  n223 = call <vilib>:"WPI_MotorControlRefNum Registry Get.vi"("refnum name"=w18) -> ("MotorControlDevRef"=w9:T1)  [unwired: 9 in, 1 out]
  n224 = call <vilib>:"WPI_MotorControlRefNum Registry Get.vi"("refnum name"=w13) -> ("MotorControlDevRef"=w10:T1)  [unwired: 9 in, 1 out]
  n225 = call <vilib>:"WPI_MotorControlRefNum Registry Get.vi"("refnum name"=w12) -> ("MotorControlDevRef"=w11:T1)  [unwired: 9 in, 1 out]
  n226 = while {
    shift-right: [w320] -> _
    shift-left: w69 -> [w320]
    shift-right: [w317] -> _
    shift-left: _ -> [w318]
    tunnel: w39 -> [w316]
    tunnel: [w308] -> _
    tunnel: w38 -> [w308]
    tunnel: w34 -> [w315]
    tunnel: w33 -> [w314]
    tunnel: w32 -> [w313]
    tunnel: w27 -> [w312]
    tunnel: w26 -> [w311]
    tunnel: w25 -> [w310]
    tunnel: w24 -> [w309]
    tunnel: w14 -> [w307]
    tunnel: w11 -> [w306]
    tunnel: w10 -> [w305]
    tunnel: w9 -> [w304]
    tunnel: w8 -> [w303]
    tunnel: w6 -> [w302]
    tunnel: w3 -> [w301]
    stop <- FALSE stop-if-true
    n227 = Tick Count (ms)() -> (millisecond timer value=w317:u32)
    n228 = Subtract(x=w317, y=w318) -> (x-y=→"Sensor Loop (ms)":u32)
    n229 = call "GetSensorValues.vi"("Ref_BuiltInAccelerometer"=w302, "Rear Prox Sensor"=w315, "Right Prox Sensor"=w314, "Left Prox Sensor"=w313, "Upper Pressure Transducer"=w312, "Ref_Compressor"=w308, "Front-Right Prox Sensor"=w311, "Ref_ElevatorEncoder"=w316, "Front-Left Prox Sensor"=w310, "Ref_ElevatorLimitSwitches"=w307, "Tank Pressure Transducer"=w309, "Ground Prox Sensor"=w301, "Ref_Drive 1R"=w306, "Ref_Drive 2R"=w305, "Ref_Drive 3L"=w304, "Ref_Drive 4L"=w303) -> ()  [unwired: 12 in]
    n230 = Wait (ms)(milliseconds to wait=u32 40) -> ()  [unwired: 1 out]
  }
